vi "Instrument Class Paths.vi"(7 "instrument":T1=enum."PPMS 1") -> (3 "Instrument Path":path[](array[path]))   [LabVIEW 2016, in "Control Experiment.lvclass"]
uses:
  Control Experiment.lvclass
  Typedefs/Instrument--enum.ctl
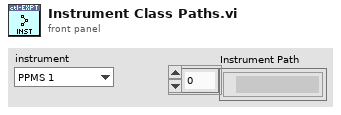
[diagram p1: front panel]
types:
  T1 = typedef "Control Experiment.lvclass/Instrument--enum.ctl" = enum16{"----- AFM/EBL -----", "AGILENT", "CYPHER", "Gemini2", "JEOL", "MFP3D", "----- Cryostat -----", "CF900", "DR200", "MNK", "PPMS 1", "PPMS 2", "PPMS 3", "----- Optics -----", "THz 1 (Element 2/Montana)", "THz 2 (Tsunami/Janis)"}
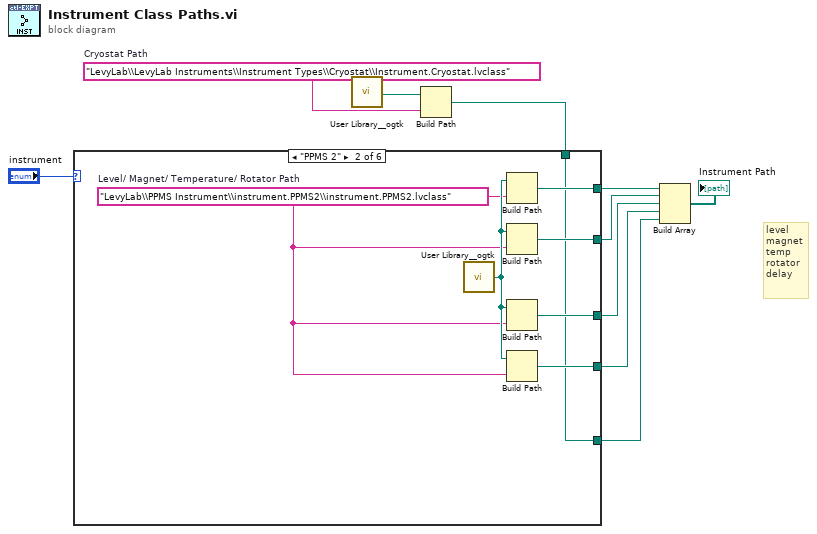
[diagram p0: block diagram]
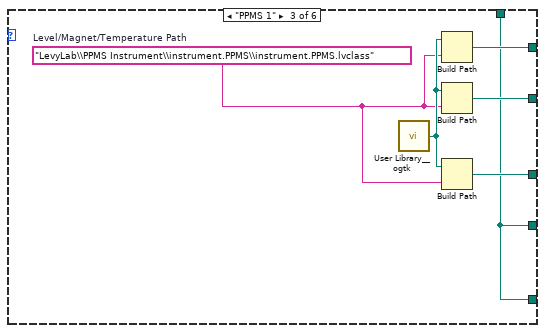
[diagram p3: hidden frame]
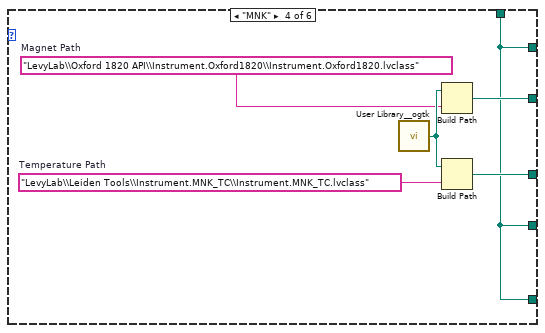
[diagram p4: hidden frame]
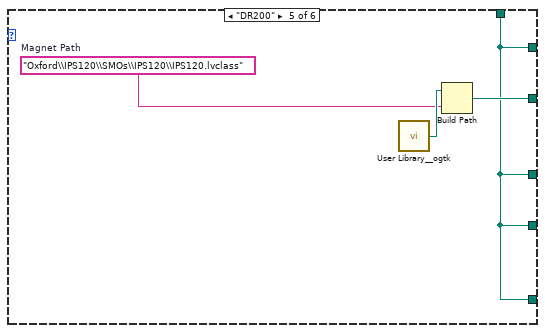
[diagram p5: hidden frame]
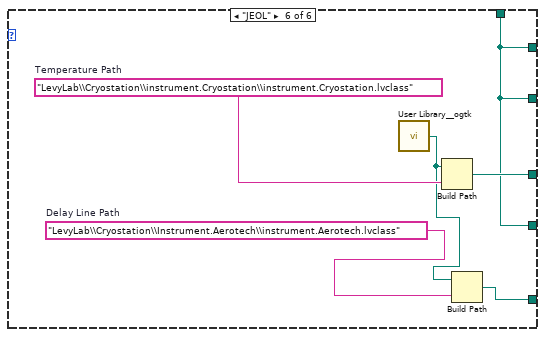
[diagram p6: hidden frame]
diagram:
  w8 = "LevyLab\\LevyLab Instruments\\Instrument Types\\Cryostat\\Instrument.Cryostat.lvclass"  # Cryostat Path
  # "level\nmagnet\ntemp\nrotator\ndelay"
  n1 = call <userlib>:"User Library__ogtk.vi"() -> ("User Library (+ Relative)"=w9:path)  [unwired: 1 in]
  n2 = Build Path(base path=w9, name or relative path=w8) -> (appended path=w7:path)
  n3 = case shown="\"PPMS 2\"" "instrument" {
    tunnel: [w11 w18 w24 w29 w31 w40] -> w3
    tunnel: [w11 w17 w23 w28 w34 w39] -> w4
    tunnel: [w11 w16 w19 w25 w31 w39] -> w2
    tunnel: [w11 w15 w22 w25 w31 w39] -> w6
    tunnel: w7 -> [w11 w12 w19 w25 w31 w39]
    tunnel: [w11 w12 w19 w25 w31 w36] -> w1
    frame Default {
    }
    frame "PPMS 2" {
      w13 = "LevyLab\\PPMS Instrument\\instrument.PPMS2\\instrument.PPMS2.lvclass"  # Level/ Magnet/ Temperature/ Rotator Path
      n4 = call <userlib>:"User Library__ogtk.vi"() -> ("User Library (+ Relative)"=w14:path)  [unwired: 1 in]
      n5 = Build Path(base path=w14, name or relative path=w13) -> (appended path=w15:path)
      n6 = Build Path(base path=w14, name or relative path=w13) -> (appended path=w17:path)
      n7 = Build Path(base path=w14, name or relative path=w13) -> (appended path=w18:path)
      n8 = Build Path(base path=w14, name or relative path=w13) -> (appended path=w16:path)
    }
    frame "PPMS 1" {
      w20 = "LevyLab\\PPMS Instrument\\instrument.PPMS\\instrument.PPMS.lvclass"  # Level/Magnet/Temperature Path
      n9 = call <userlib>:"User Library__ogtk.vi"() -> ("User Library (+ Relative)"=w21:path)  [unwired: 1 in]
      n10 = Build Path(base path=w21, name or relative path=w20) -> (appended path=w22:path)
      n11 = Build Path(base path=w21, name or relative path=w20) -> (appended path=w23:path)
      n12 = Build Path(base path=w21, name or relative path=w20) -> (appended path=w24:path)
    }
    frame "MNK" {
      w26 = "LevyLab\\Oxford 1820 API\\Instrument.Oxford1820\\Instrument.Oxford1820.lvclass"  # Magnet Path
      w30 = "LevyLab\\Leiden Tools\\Instrument.MNK_TC\\Instrument.MNK_TC.lvclass"  # Temperature Path
      n13 = call <userlib>:"User Library__ogtk.vi"() -> ("User Library (+ Relative)"=w27:path)  [unwired: 1 in]
      n14 = Build Path(base path=w27, name or relative path=w26) -> (appended path=w28:path)
      n15 = Build Path(base path=w27, name or relative path=w30) -> (appended path=w29:path)
    }
    frame "DR200" {
      w32 = "Oxford\\IPS120\\SMOs\\IPS120\\IPS120.lvclass"  # Magnet Path
      n16 = call <userlib>:"User Library__ogtk.vi"() -> ("User Library (+ Relative)"=w33:path)  [unwired: 1 in]
      n17 = Build Path(base path=w33, name or relative path=w32) -> (appended path=w34:path)
    }
    frame "JEOL" {
      w35 = "LevyLab\\Cryostation\\Instrument.Aerotech\\instrument.Aerotech.lvclass"  # Delay Line Path
      w38 = "LevyLab\\Cryostation\\instrument.Cryostation\\instrument.Cryostation.lvclass"  # Temperature Path
      n18 = call <userlib>:"User Library__ogtk.vi"() -> ("User Library (+ Relative)"=w37:path)  [unwired: 1 in]
      n19 = Build Path(base path=w37, name or relative path=w38) -> (appended path=w40:path)
      n20 = Build Path(base path=w37, name or relative path=w35) -> (appended path=w36:path)
    }
  }
  n21 = Build Array(w6, w4, w3, w2, w1) -> (→"Instrument Path":path[])
